vi "My OWn PID.vi"(8 "Current Input":dbl, 11 "Wanted End":dbl) -> (3 "Output":dbl)   [LabVIEW 2017]
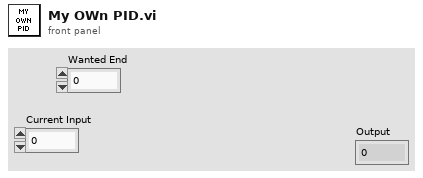
[diagram p1: front panel]
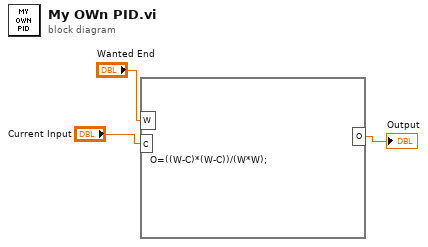
[diagram p0: block diagram]
diagram:
  n1 = formula code="O=((W-C)*(W-C))/(W*W);"("W"="Wanted End", "C"="Current Input") -> ("O"=→"Output":dbl)
